vi "Write Last Header Class.vi"(8 "error in (no error)":errorcluster, 10 "Simulated_Header.lvclass":refnum<class "Simulated_Header.lvclass">, 11 "Save Image in":refnum<class "Save Image.lvclass">) -> (0 "error out":errorcluster, 3 "Save Image out":refnum<class "Save Image.lvclass">)   [LabVIEW 2018, in "Save Image.lvclass"]
uses:
  Save Image.lvclass
  Simulated_Header/Simulated_Header.lvclass
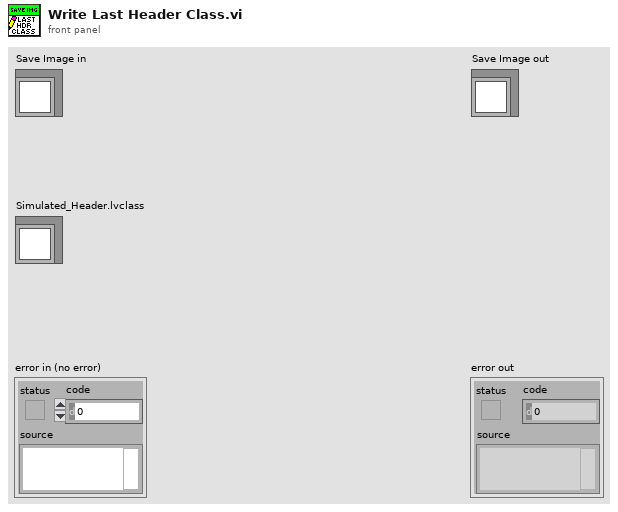
[diagram p1: front panel]
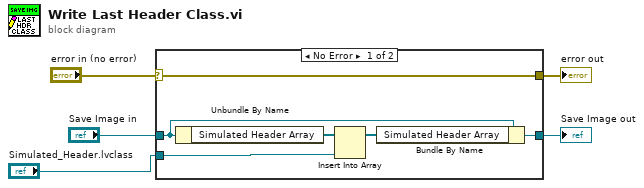
[diagram p0: block diagram]
diagram:
  n1 = case shown="No Error" "error in (no error)" {
    selector: "error in (no error)" -> [w11 w12]
    tunnel: [w11 w12] -> w4
    tunnel: [w10 w13] -> w2
    tunnel: "Save Image in" -> [w9 w13]
    tunnel: "Simulated_Header.lvclass" -> [w6 _]
    frame No Error {
      n2 = Unbundle By Name(w9) -> ("Simulated Header Array"=w8:refnum<class "Simulated_Header.lvclass">[])
      n3 = Insert Into Array(array=w8, new element=w6) -> (w7:refnum<class "Simulated_Header.lvclass">[])  [unwired: 1 in]
      n4 = Bundle By Name(cluster=w9, "Simulated Header Array"=w7) -> (w10:refnum<class "Save Image.lvclass">)
    }
    frame Error {
    }
  }
  "error out" <- w4
  "Save Image out" <- w2
